vi "Voltage sweep.vi"() -> ()   [LabVIEW 2017]
doc: "This example shows how to create, run a script and query the script output data."
uses:
  <instrlib>/Keithley 2600 Series/Keithley 2600 Series.lvlib
panel:
  out "PV":T1(graph)
  out "PCE(a.u.)":dbl
  in  "Pin(W/cm^2)":dbl=0.1
  out "FF(a.u.)":dbl
  out "Jsc(A/cm^2)":dbl
  in  "Area(cm^2)":dbl=0.085
  out "Voc(V)":dbl
  out "Ioc(A)":dbl
  out "Vsc(V)":dbl
  out "Isc(A)":dbl
  out "IMP(A)":dbl
  out "VMP(V)":dbl
  out "PMP(W)":dbl
  out "output array":string[][](array[string])
  in  "SweepSetting":T2={"CurrentLimit(A)"=0.1, "Start Voltage(V)"=-0.5, "Stop Voltage(V)"=0.9, "Dwell Time(mS)"=150.0, "NumPoint"=75.0} {"NumPoint" min=1.0 max=75.0 step=1.0; "Dwell Time(mS)" min=50.0 max=150.0; "Stop Voltage(V)" min=-200.0 max=200.0; "Start Voltage(V)" min=-200.0 max=200.0; "CurrentLimit(A)" min=1e-09 max=1.5}
  out "IV":cluster{"array type (2D Dbl)":dbl[], dbl[]}(graph)
  in  "USB COM Port":refnum<visa-resource-name>="COM3"
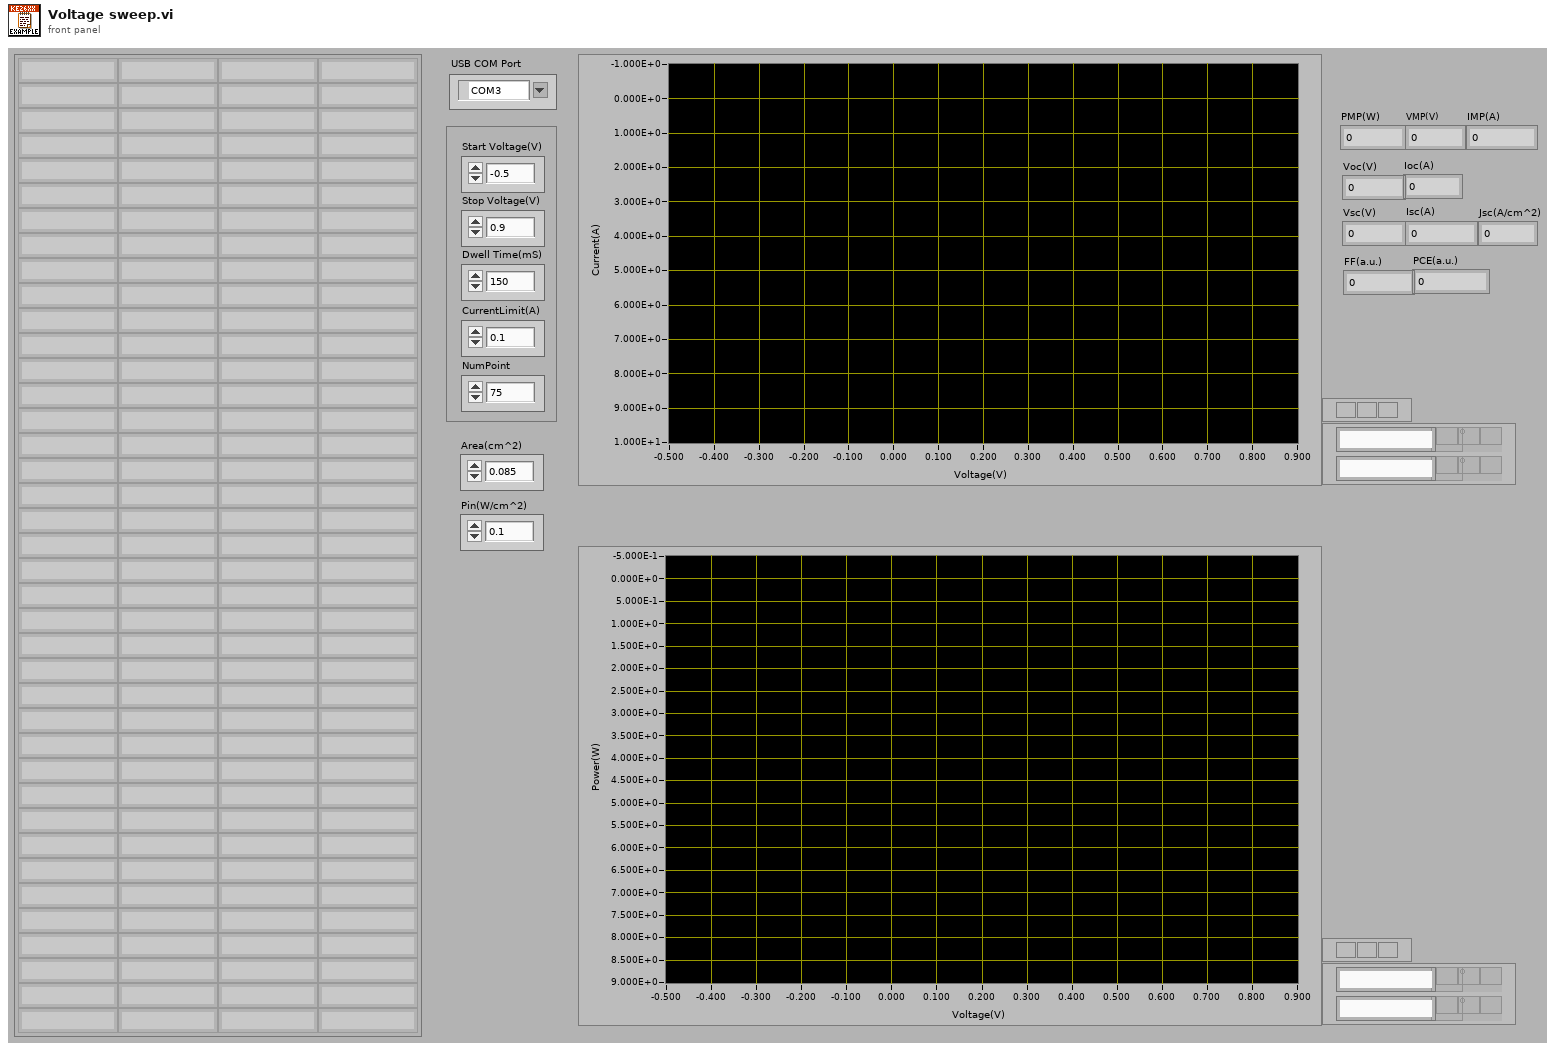
[diagram p1: front panel]
types:
  T1 = cluster{"array type (2D Dbl)":dbl[], "array type (2D Dbl)":dbl[]}
  T2 = cluster{"CurrentLimit(A)":dbl, "Start Voltage(V)":dbl, "Stop Voltage(V)":dbl, "Dwell Time(mS)":dbl, "NumPoint":dbl}
  T3 = cluster{"Baud Rate":u32, "Parity":u16, "Data Bits":u16, "Stop Bits":u16, "Flow Control":u16}
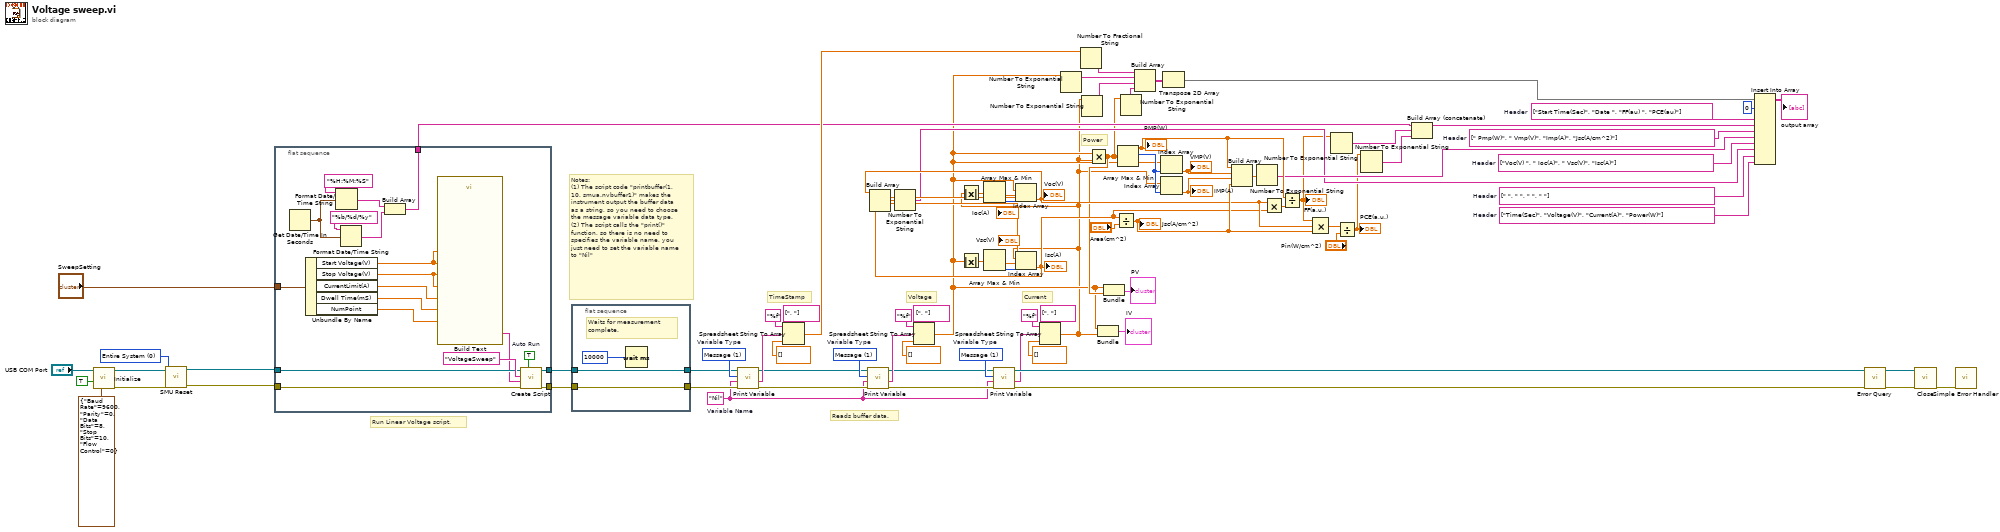
[diagram p0: block diagram]
diagram:
  w7 = 0 items=["Entire System", "Local Group", "Local Node", "Remote Node", "Source Measure Unit Channel A", "Source Measure Unit Channel B", "LAN", "TSP Net", "TSP Link", "Timer"] ("Reset Module (0: Entire System)")
  w19 = string[] ["Voc(V) ", " Ioc(A)", " Vsc(V)", "Isc(A)"]  # Header
  w20 = string[] [" Pmp(W)", " Vmp(V)", "Imp(A)", "Jsc(A/cm^2)"]  # Header
  w16 = string[] ["Time(Sec)", "Voltage(V)", "Current(A)", "Power(W)"]  # Header
  w17 = string[] [" ", " ", " ", " "]  # Header
  w33 = string[] ["Start Time(Sec)", "Date ", "FF(au) ", "PCE(au)"]  # Header
  w64 = 1 items=["Number", "Message"]  # Variable Type
  w65 = 1 items=["Number", "Message"]  # Variable Type
  w84 = 1 items=["Number", "Message"]  # Variable Type
  w53 = "Nil"  # Variable Name
  # "Power"
  # "Current"
  # "Voltage"
  # "TimeStamp"
  # "Reads buffer data."
  # "Notes: \n(1) The script code \"printbuffer(1, 10, smua.nvbuffer1)\" makes the instrument output the buffer data as a string, so you need to choose the message variable data type.\n(2) The script calls the \"print()\" function, so there is no need to specifies the variable name, you just need to set the variable name to \"Nil\""
  # "Run Linear Voltage script."
  n1 = call <instrlib>:"Initialize.vi"("Serial Configuration"=T3 {"Baud Rate"=9600, "Parity"=0, "Data Bits"=8, "Stop Bits"=10, "Flow Control"=0}, "Reset (True)"=TRUE, "VISA resource name"="USB COM Port") -> ("error out"=w8:errorcluster, "VISA resource name out"=w11:refnum<visa-resource-name>)  [unwired: 7 in]
  n2 = call <instrlib>:"SMU Reset.vi"("error in (no error)"=w8, "Reset Module (0: Entire System)"=w7, "VISA resource name"=w11) -> ("error out"=w9:errorcluster, "VISA resource name out"=w10:refnum<visa-resource-name>)  [unwired: 7 in]
  n3 = flat-sequence {
    tunnel: [w101] -> w83
    tunnel: [w100] -> w82
    tunnel: w10 -> [w99]
    tunnel: w9 -> [w98]
    tunnel: "SweepSetting" -> [w96]
    tunnel: [w90] -> w34
    frame #0 {
      w102 = TRUE  # Auto Run
      n4 = Get Date/Time In Seconds() -> (seconds since 1Jan1904=w91:timestamp)
      n5 = Unbundle By Name(w96) -> ("Start Voltage(V)"=w89:dbl, "Stop Voltage(V)"=w88:dbl, "CurrentLimit(A)"=w87:dbl, "Dwell Time(mS)"=w86:dbl, "NumPoint"=w85:dbl)
      n6 = Format Date/Time String(time format string (%c)="%H:%M:%S", seconds (now)=w91) -> (date/time string=w94:string)  [unwired: 1 out]
      n7 = Format Date/Time String(time format string (%c)="%b/%d/%y", seconds (now)=w91) -> (date/time string=w92:string)  [unwired: 1 out]
      n8 = Build Array(w94, w92) -> (w90:string[])
      n9 = call "Build Text"("numPoints"=w85, "stopV1"=w88, "limitI"=w87, "stopV"=w88, "startV"=w89, "startV1"=w89, "dwellTime"=w86) -> ("Result"=w97:string)  [unwired: 7 in, 1 out]
      n10 = call <instrlib>:"Create Script.vi"("Auto Run (F: Disable)"=w102, "error in (no error)"=w98, "Source Code"=w97, "Script Variable"="VoltageSweep" ("Script Variable (myScript)"), "VISA resource name"=w99) -> ("error out"=w100:errorcluster, "VISA resource name out"=w101:refnum<visa-resource-name>)  [unwired: 5 in]
    }
  }
  n11 = flat-sequence {
    tunnel: w83 -> [w104]
    tunnel: w82 -> [w105]
    tunnel: [w105] -> w80
    tunnel: [w104] -> w81
    frame #0 {
      # "Waits for measurement complete."
      n12 = Wait (ms)(milliseconds to wait=10000 ("Temp Delay")) -> ()  [unwired: 1 out]
    }
  }
  n13 = call <instrlib>:"Print Variable.vi"("error in (no error)"=w80, "Variable Name"=w53, "Variable Type (0: Number)"=w84, "VISA resource name"=w81) -> ("error out"=w61:errorcluster, "Message"=w70:string, "VISA resource name out"=w62:refnum<visa-resource-name>)  [unwired: 4 in, 1 out]
  n14 = Spreadsheet String To Array(delimiter (Tab)=string[] [", "], format string="%f", spreadsheet string=w70, array type (2D Dbl)=dbl[] []) -> (array=w47:dbl[])
  n15 = call <instrlib>:"Print Variable.vi"("error in (no error)"=w61, "Variable Name"=w53, "Variable Type (0: Number)"=w65, "VISA resource name"=w62) -> ("error out"=w59:errorcluster, "Message"=w69:string, "VISA resource name out"=w60:refnum<visa-resource-name>)  [unwired: 4 in, 1 out]
  n16 = Spreadsheet String To Array(delimiter (Tab)=string[] [", "], format string="%f", spreadsheet string=w69, array type (2D Dbl)=dbl[] []) -> (array=w5:dbl[])
  n17 = Absolute Value(x=w5) -> (abs(x)=w43:dbl[])
  n18 = Array Max & Min(array=w43) -> (min value=w22:dbl, min index (indices)=w42:i32)  [unwired: 2 out]
  "Vsc(V)" <- w22
  n19 = call <instrlib>:"Print Variable.vi"("error in (no error)"=w59, "Variable Name"=w53, "Variable Type (0: Number)"=w64, "VISA resource name"=w60) -> ("error out"=w57:errorcluster, "Message"=w55:string, "VISA resource name out"=w58:refnum<visa-resource-name>)  [unwired: 4 in, 1 out]
  n20 = Spreadsheet String To Array(delimiter (Tab)=string[] [", "], format string="%f", spreadsheet string=w55, array type (2D Dbl)=dbl[] []) -> (array=w4:dbl[])
  n21 = Absolute Value(x=w4) -> (abs(x)=w40:dbl[])
  n22 = Array Max & Min(array=w40) -> (min value=w23:dbl, min index (indices)=w41:i32)  [unwired: 2 out]
  "Ioc(A)" <- w23
  n23 = Index Array(array=w5, index=w41) -> (element=w24:dbl)
  "Voc(V)" <- w24
  n24 = Index Array(array=w4, index=w42) -> (element=w21:dbl)
  "Isc(A)" <- w21
  n25 = Build Array(w24, w23, w22, w21) -> (w25:dbl[])
  n26 = Number To Exponential String(number=w25) -> (E-format string=w18:string[])  [unwired: 3 in]
  n27 = Number To Exponential String(number=w5) -> (E-format string=w50:string[])  [unwired: 3 in]
  n28 = Number To Fractional String(number=w47) -> (F-format string=w51:string[])  [unwired: 3 in]
  n29 = Number To Exponential String(number=w4) -> (E-format string=w45:string[])  [unwired: 3 in]
  n30 = Multiply(x=w5, y=w4) -> (x*y=w6:dbl[])
  n31 = Bundle("array type (2D Dbl)"=w5, "array type (2D Dbl)"=w4) -> (→"IV":T1)  [unwired: 1 in]
  n32 = Bundle("array type (2D Dbl)"=w5, w6) -> (→"PV":cluster{"array type (2D Dbl)":dbl[], dbl[]})  [unwired: 1 in]
  n33 = Divide(x=w21, y="Area(cm^2)") -> (x/y=w28:dbl)
  "Jsc(A/cm^2)" <- w28
  n34 = Array Max & Min(array=w6) -> (max value=w31:dbl, max index (indices)=w44:i32)  [unwired: 2 out]
  "PMP(W)" <- w31
  n35 = Number To Exponential String(number=w6) -> (E-format string=w35:string[])  [unwired: 3 in]
  n36 = Build Array(w51, w50, w45, w35) -> (w52:string[][])
  n37 = Index Array(array=w5, index=w44) -> (element=w30:dbl)
  "VMP(V)" <- w30
  n38 = Index Array(array=w4, index=w44) -> (element=w29:dbl)
  "IMP(A)" <- w29
  n39 = Transpose 2D Array(2D array=w52) -> (transposed array=w49:string[][])
  n40 = Build Array(w31, w30, w29, w28) -> (w27:dbl[])
  n41 = Number To Exponential String(number=w27) -> (E-format string=w26:string[])  [unwired: 3 in]
  n42 = Multiply(x=w21, y=w24) -> (x*y=w38:dbl)
  n43 = Divide(x=w31, y=w38) -> (x/y=w14:dbl)
  "FF(a.u.)" <- w14
  n44 = Compound Arithmetic op=MULTIPLY(w14, w24, w28) -> (w37:dbl)
  n45 = Number To Exponential String(number=w14) -> (E-format string=w13:string)  [unwired: 3 in]
  n46 = Divide(x=w37, y="Pin(W/cm^2)") -> (x/y=w15:dbl)
  "PCE(a.u.)" <- w15
  n47 = Number To Exponential String(number=w15) -> (E-format string=w12:string)  [unwired: 3 in]
  n48 = Build Array (concatenate)(w34, w13, w12) -> (w32:string[])
  n49 = Insert Into Array(array=w49, index (row)=0, new element #1=w33, new element #2=w32, new element #3=w20, new element #4=w26, new element #5=w19, new element #6=w18, new element #7=w17, new element #8=w16) -> (→"output array":string[][])  [unwired: 1 in]
  n50 = call <instrlib>:"Error Query.vi"("error in (no error)"=w57, "VISA resource name"=w58) -> ("error out"=w78:errorcluster, "VISA resource name out"=w79:refnum<visa-resource-name>)  [unwired: 6 in, 2 out]
  n51 = call <instrlib>:"Close.vi"("error in (no error)"=w78, "VISA resource name"=w79) -> ("error out"=w3:errorcluster)  [unwired: 9 in]
  n52 = call <vilib>:"Simple Error Handler.vi"("error in (no error)"=w3) -> ()  [unwired: 4 in, 5 out]
